vi "Do Obstacle Avoidance.vi"(5 "Target Distance":dbl=250.0, 8 "Wall Left?":bool=TRUE, 10 "Bot Angle (rad)":dbl=0.024476546476243494, 11 "Lidar Data (mm, rad)":cluster{dbl[], dbl[]}(graph)={[259.0, 261.0, 264.0, 264.0, 264.0, 261.0, 258.0, 258.0, 254.99999999999997, 255.0, 255.0, 253.0, 252.99999999999997, 260.0, 260.0, 260.0, 260.0, 260.0, 260.0, 257.0, 260.0, 263.0, 263.0, 262.0, 262.0, 260.0, 260.0, 262.0, 260.0, 263.0, 263.0, 256.0, 255.99999999999997, 256.0, 256.0, 260.0, 262.0, 262.0, 264.99999999999994, 262.0, 265.0, 265.0, 265.0, 265.0, 265.0, 265.0, 262.0, 262.0, 266.0, 266.0, 266.0, 266.0, 261.0, 259.0, 259.0, 259.0, 259.0, 261.0, 264.0, 261.0, 262.0, 262.0, 260.0, 260.0, 262.0, 262.0, 262.0, 262.0, 264.0, 263.0, 263.0, 272.0, 272.0, 272.0, 272.0, 272.0, 272.0, 272.0, 272.0, 272.0, 271.0, 270.0, 270.0, 269.0, 269.0, 269.0, 275.0, 276.0, 276.0, 277.0, 275.0, 277.0, 277.0, 277.0, 281.0, 281.0, 281.0, 284.0, 281.0, 281.0, 282.0, 282.0, 282.0, 283.0, 283.0, 295.99999999999994, 296.0, 291.00000000000006, 291.0, 291.0, 290.0, 291.0, 291.0, 291.0, 291.0, 300.0, 299.0, 299.0, 300.0, 307.0, 304.0, 311.0, 311.0, 308.0, 308.0, 308.0, 308.0, 308.0, 313.0, 319.0, 319.0, 322.0, 323.0, 326.0, 324.0, 326.0, 326.0, 329.0, 331.0, 336.99999999999994, 338.0, 338.0, 338.0, 338.0, 338.0, 338.0, 345.00000000000006, 350.0, 348.0, 349.99999999999994, 350.0, 351.0, 355.0, 358.0, 358.99999999999994, 358.0, 359.0, 367.0, 370.0, 367.00000000000006, 370.0, 372.0, 379.0, 379.0, 385.0, 387.0, 388.0, 394.0, 406.0, 406.99999999999994, 407.0, 408.0, 417.00000000000006, 417.0, 417.0, 417.0, 424.0, 428.0, 427.99999999999994, 428.99999999999994, 432.0, 432.0, 443.00000000000006, 452.0, 452.0, 454.0, 462.0, 464.00000000000006, 464.0, 464.00000000000006, 470.0, 480.99999999999994, 484.0, 494.0, 498.00000000000006, 499.00000000000006, 509.00000000000006, 508.99999999999994, 514.0, 521.0, 522.0, 533.0, 545.0, 546.0, 551.0, 555.0, 557.0, 567.0, 570.0, 573.0, 595.0, 606.0, 617.0, 619.0, 638.0, 643.0, 650.0, 667.0, 734.0, 734.0, 733.9999999999999, 728.0000000000001, 725.0, 720.0, 716.0, 713.0000000000001, 713.0, 715.0, 715.0, 714.9999999999999, 715.0, 698.0, 698.0, 698.0, 699.0000000000001, 699.0, 699.0, 693.0, 693.0, 693.0, 697.0, 697.0, 697.0, 688.0, 685.0, 684.9999999999999, 680.0, 684.0, 684.0, 684.0, 675.0, 683.0, 680.0, 680.0, 671.0, 670.0, 668.0, 667.9999999999999, 668.0, 668.0, 662.0, 668.0, 668.0, 669.9999999999999, 670.0, 670.0, 660.0, 659.0, 659.0, 660.0, 660.0, 662.0, 662.0, 661.0, 661.0, 661.0, 655.0, 655.0, 655.0, 653.0, 655.0, 654.0, 666.0, 654.0, 666.0, 654.0, 653.0, 647.0, 647.0, 647.0, 647.0, 651.0, 652.0, 653.0, 654.0, 654.0, 654.0, 654.0, 648.0, 648.0, 654.0, 650.0, 657.0, 657.0, 656.0, 654.0, 656.0, 656.0, 656.0, 654.0, 654.0, 654.0, 654.0, 654.0, 656.0, 656.0, 658.0, 656.0, 658.0, 656.0, 653.0, 650.0, 653.0, 652.9999999999999, 653.0, 659.0, 666.0, 666.0, 666.0000000000001, 670.0, 670.0, 670.0, 669.0000000000001, 670.0, 669.0, 670.0, 670.0, 678.0, 671.9999999999999, 678.0, 674.0, 678.0000000000001, 677.0, 683.0, 677.0, 677.0, 677.0, 688.0, 710.0, 782.0, 880.9999999999999, 840.0, 881.0, 881.0, 817.0, 896.0, 848.0, 848.0, 827.0, 815.0, 748.0, 748.0, 748.0, 754.0, 756.0, 68.0, 68.0, 68.0], [-1.7446474827552692, -1.7385115596037266, -1.732375636452184, -1.7262397133006415, -1.7201037901490988, -1.7139678669975562, -1.7078319438460137, -1.7016960206944711, -1.6955600975429286, -1.689424174391386, -1.6832882512398435, -1.677152328088301, -1.6710164049367584, -1.6648804817852159, -1.658744558633673, -1.6526086354821306, -1.646472712330588, -1.6403367891790455, -1.634200866027503, -1.6280649428759604, -1.6219290197244178, -1.6157930965728753, -1.6096571734213327, -1.6035212502697902, -1.5973853271182477, -1.591249403966705, -1.5851134808151623, -1.5789775576636198, -1.5728416345120773, -1.566705711360535, -1.5605697882089924, -1.5544338650574498, -1.5482979419059073, -1.5421620187543645, -1.536026095602822, -1.5298901724512795, -1.523754249299737, -1.5176183261481944, -1.5114824029966518, -1.5053464798451093, -1.4992105566935667, -1.4930746335420242, -1.4869387103904816, -1.480802787238939, -1.4746668640873963, -1.4685309409358538, -1.4623950177843112, -1.4562590946327687, -1.4501231714812262, -1.4439872483296836, -1.437851325178141, -1.4317154020265985, -1.425579478875056, -1.4194435557235134, -1.413307632571971, -1.4071717094204281, -1.4010357862688856, -1.394899863117343, -1.3887639399658005, -1.382628016814258, -1.3764920936627154, -1.3703561705111729, -1.3642202473596303, -1.3580843242080878, -1.3519484010565452, -1.3458124779050025, -1.33967655475346, -1.3335406316019174, -1.3274047084503748, -1.3212687852988323, -1.3151328621472897, -1.3089969389957472, -1.3028610158442047, -1.2967250926926621, -1.2905891695411196, -1.284453246389577, -1.2783173232380343, -1.2721814000864917, -1.2660454769349492, -1.2599095537834066, -1.253773630631864, -1.2476377074803215, -1.241501784328779, -1.2353658611772365, -1.229229938025694, -1.2230940148741514, -1.2169580917226088, -1.210822168571066, -1.2046862454195235, -1.198550322267981, -1.1924143991164384, -1.1862784759648959, -1.1801425528133533, -1.1740066296618108, -1.1678707065102683, -1.1617347833587257, -1.1555988602071832, -1.1494629370556404, -1.1433270139040979, -1.1371910907525553, -1.1310551676010128, -1.1249192444494702, -1.1187833212979277, -1.1126473981463851, -1.1065114749948426, -1.1003755518433, -1.0942396286917575, -1.088103705540215, -1.0819677823886722, -1.0758318592371297, -1.069695936085587, -1.0635600129340446, -1.057424089782502, -1.0512881666309595, -1.045152243479417, -1.0390163203278744, -1.0328803971763318, -1.0267444740247893, -1.0206085508732468, -1.014472627721704, -1.0083367045701614, -1.002200781418619, -0.9960648582670764, -0.9899289351155338, -0.9837930119639913, -0.9776570888124487, -0.9715211656609062, -0.9653852425093635, -0.959249319357821, -0.9531133962062782, -0.9469774730547359, -0.9408415499031934, -0.9347056267516507, -0.9285697036001082, -0.9224337804485656, -0.9162978572970231, -0.9101619341454805, -0.9040260109939379, -0.8978900878423952, -0.8917541646908528, -0.8856182415393102, -0.8794823183877678, -0.8733463952362251, -0.8672104720846825, -0.8610745489331402, -0.8549386257815974, -0.8488027026300549, -0.8426667794785123, -0.8365308563269697, -0.8303949331754271, -0.8242590100238846, -0.818123086872342, -0.8119871637207995, -0.8058512405692568, -0.7997153174177143, -0.793579394266172, -0.7874434711146292, -0.7813075479630864, -0.775171624811544, -0.7690357016600015, -0.7628997785084586, -0.7567638553569163, -0.7506279322053737, -0.7444920090538312, -0.7383560859022886, -0.732220162750746, -0.7260842395992034, -0.7199483164476609, -0.7138123932961183, -0.7076764701445758, -0.7015405469930333, -0.6954046238414906, -0.689268700689948, -0.6831327775384055, -0.676996854386863, -0.6708609312353204, -0.6647250080837778, -0.6585890849322352, -0.6524531617806927, -0.64631723862915, -0.6401813154776076, -0.6340453923260647, -0.6279094691745224, -0.6217735460229799, -0.6156376228714373, -0.6095016997198948, -0.6033657765683523, -0.5972298534168096, -0.591093930265267, -0.5849580071137245, -0.5788220839621819, -0.5726861608106395, -0.5665502376590967, -0.5604143145075542, -0.5542783913560116, -0.5481424682044691, -0.5420065450529266, -0.5358706219013839, -0.5297346987498412, -0.5235987755982987, -0.5174628524467563, -0.5113269292952137, -0.5051910061436712, -0.4990550829921286, -0.492919159840586, -0.48678323668904344, -0.4806473135375009, -0.47451139038595824, -0.46837546723441575, -0.4622395440828731, -0.4561036209313306, -0.44996769777978807, -0.44383177462824547, -0.4376958514767028, -0.43155992832516044, -0.4254240051736178, -0.41928808202207524, -0.4131521588705326, -0.4070162357189901, -0.40088031256744755, -0.39474438941590495, -0.38860846626436246, -0.38247254311281986, -0.3763366199612773, -0.3702006968097348, -0.3640647736581921, -0.35792885050664963, -0.351792927355107, -0.3456570042035645, -0.33952108105202194, -0.3333851579004794, -0.3272492347489368, -0.32111331159739426, -0.31497738844585166, -0.3088414652943091, -0.3027055421427665, -0.29656961899122397, -0.2904336958396814, -0.2842977726881388, -0.2781618495365963, -0.27202592638505374, -0.2658900032335112, -0.2597540800819686, -0.25361815693042605, -0.2474822337788835, -0.24134631062734088, -0.23521038747579834, -0.2290744643242557, -0.2229385411727132, -0.21680261802117062, -0.21066669486962808, -0.2045307717180855, -0.19839484856654294, -0.19225892541500036, -0.1861230022634578, -0.17998707911191522, -0.17385115596037265, -0.16771523280883013, -0.16157930965728756, -0.15544338650574496, -0.14930746335420234, -0.14317154020265982, -0.13703561705111728, -0.1308996938995747, -0.12476377074803216, -0.11862784759648957, -0.11249192444494702, -0.10635600129340447, -0.10022007814186189, -0.09408415499031934, -0.08794823183877676, -0.0818123086872342, -0.07567638553569163, -0.06954046238414907, -0.06340453923260649, -0.05726861608106395, -0.05113269292952138, -0.044996769777978805, -0.03886084662643624, -0.03272492347489367, -0.026589000323351118, -0.02045307717180855, -0.014317154020265985, -0.008181230868723419, -0.0020453077171808547, 0.0040906154343617095, 0.010226538585904275, 0.016362461737446838, 0.022498384888989403, 0.028634308040531974, 0.03477023119207454, 0.0409061543436171, 0.04704207749515967, 0.053178000646702236, 0.0593139237982448, 0.06544984694978735, 0.07158577010132992, 0.07772169325287247, 0.08385761640441505, 0.08999353955595761, 0.09612946270750018, 0.10226538585904273, 0.10840130901058531, 0.11453723216212788, 0.12067315531367044, 0.126809078465213, 0.13294500161675557, 0.13908092476829814, 0.1452168479198407, 0.15135277107138329, 0.15748869422292583, 0.1636246173744684, 0.16976054052601097, 0.1758964636775535, 0.1820323868290961, 0.18816830998063866, 0.19430423313218123, 0.20044015628372377, 0.20657607943526632, 0.2127120025868089, 0.21884792573835146, 0.22498384888989406, 0.23111977204143658, 0.23725569519297915, 0.24339161834452172, 0.24952754149606432, 0.25566346464760686, 0.2617993877991494, 0.2679353109506919, 0.2740712341022345, 0.2802071572537771, 0.2863430804053197, 0.2924790035568622, 0.2986149267084048, 0.30475084985994744, 0.3108867730114899, 0.31702269616303236, 0.32315861931457507, 0.3292945424661176, 0.33543046561766016, 0.34156638876920276, 0.3477023119207453, 0.3538382350722879, 0.35997415822383044, 0.366110081375373, 0.3722460045269156, 0.37838192767845813, 0.3845178508300008, 0.3906537739815433, 0.3967896971330859, 0.8017606251348951, 0.8078965482864374, 0.8140324714379802, 0.8201683945895226, 0.8263043177410653, 0.8324402408926079, 0.8508480103472355, 0.856983933498778, 0.8631198566503209, 0.8692557798018633, 0.8753917029534058, 0.8815276261049484, 0.8876635492564908, 0.8937994724080335, 0.8999353955595761, 1.6669257895023968, 1.6730617126539393, 1.679197635805482]}) -> (0 "Target Angle":dbl=0.040223878073184685)   [LabVIEW 2017]
uses:
  Globals/Pose.vi
  <vilib>/robotics/Obstacle Avoidance/Advanced Vector Field Histogram/NI_Robotics_Vector Field Histogram.lvlib
panel:
  in  "Max LIDAR Point Distance":dbl=4000.0 format="%#_13g"
  in  "Obstacle Clearance Distance":dbl=100.0 format="%#_13g"
  in  "VFH Threshold Distances":T1={"inner threshold distance"=350.0, "outer threshold distance"=360.0}
  out "LIDAR Data with Fake Wall":cluster{dbl[], dbl[]}(graph)
  # "Outputs"
  # "Inputs"
  # "Process"
  # "Thresholds need to be low enough to\nnot avoid the ramp before seeing red line"
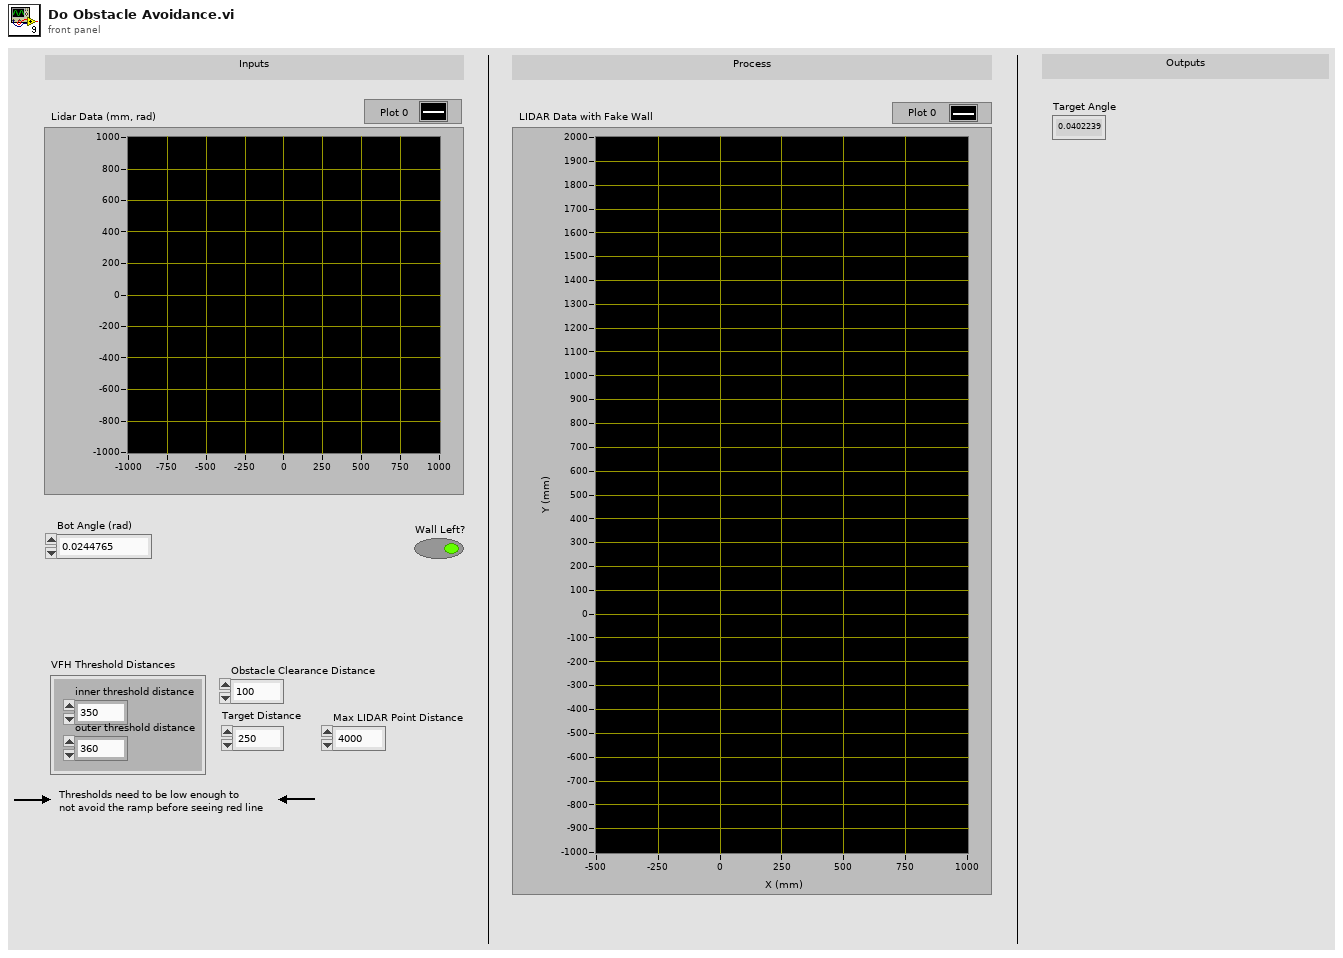
[diagram p1: front panel]
types:
  T1 = cluster{"inner threshold distance":dbl, "outer threshold distance":dbl}
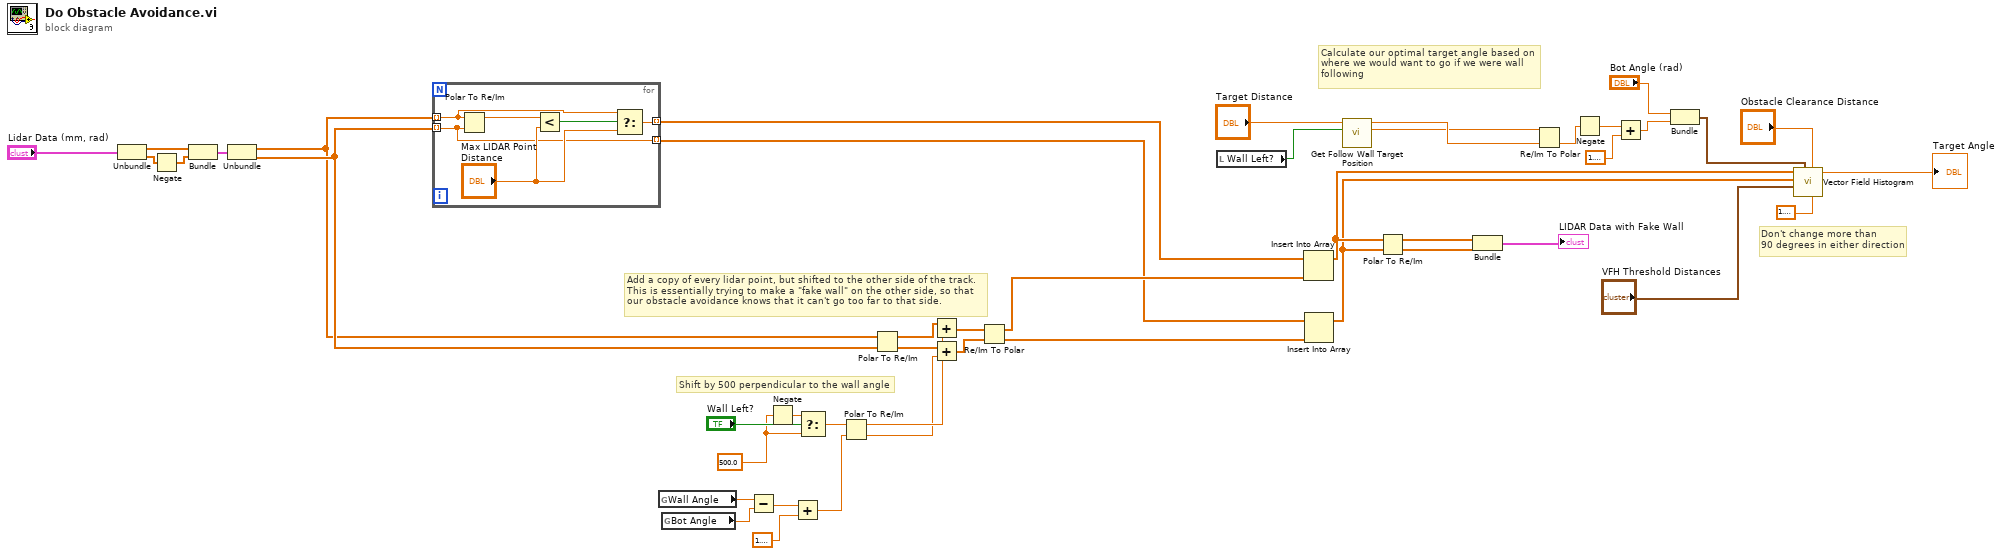
[diagram p0: block diagram]
diagram:
  w14 = 500.0 ("y")
  # "Shift by 500 perpendicular to the wall angle"
  # "Calculate our optimal target angle based on\nwhere we would want to go if we were wall\nfollowing"
  # "Don't change more than\n90 degrees in either direction"
  # "Add a copy of every lidar point, but shifted to the other side of the track.\nThis is essentially trying to make a \"fake wall\" on the other side, so that\nour obstacle avoidance knows that it can't go too far to that side."
  n1 = Unbundle("Lidar Data (mm, rad)") -> (w41:dbl[], w32:dbl[])
  n2 = Negate(x=w32) -> (-x=w31:dbl[])
  n3 = Bundle(w41, w31) -> (w40:cluster{dbl[], dbl[]})  [unwired: 1 in]
  n4 = Unbundle(w40) -> (w18:dbl[], w19:dbl[])
  n5 = for {
    tunnel: [w49] -> w20 mode=indexing
    tunnel: w19 -> [w46] mode=indexing
    tunnel: w18 -> [w47] mode=indexing
    tunnel: [w46] -> w16 mode=indexing
    n6 = Polar To Re/Im(2:w46, 3:w47) -> (1:w51:dbl)  [unwired: 1 out]
    n7 = Less?(x=w51, y="Max LIDAR Point Distance") -> (x < y?=w50:bool)
    n8 = Select(t=w47, s=w50, f="Max LIDAR Point Distance") -> (s? t:f=w49:dbl)
  }
  n9 = global read "Pose.vi" "Wall Angle"() -> (w5:dbl)
  n10 = global read "Pose.vi" "Bot Angle"() -> (w4:dbl)
  n11 = Subtract(x=w5, y=w4) -> (x-y=w3:dbl)
  n12 = Negate(x=w14) -> (-x=w21:dbl)
  n13 = Add(x=w3, y=1.5707963267948966) -> (x+y=w1:dbl)
  n14 = Select(t=w21, s="Wall Left?", f=w14) -> (s? t:f=w11:dbl)
  n15 = Polar To Re/Im(2:w1, 3:w11) -> (0:w6:dbl, 1:w7:dbl)
  n16 = Polar To Re/Im(2:w19, 3:w18) -> (0:w24:dbl[], 1:w8:dbl[])
  n17 = Add(x=w8, y=w7) -> (x+y=w9:dbl[])
  n18 = Add(x=w24, y=w6) -> (x+y=w10:dbl[])
  n19 = Re/Im To Polar(2:w10, 3:w9) -> (0:w22:dbl[], 1:w23:dbl[])
  n20 = local read "Wall Left?"() -> (w15:bool)
  n21 = Insert Into Array(array=w20, new element=w23) -> (w34:dbl[])  [unwired: 1 in]
  n22 = Insert Into Array(array=w16, new element=w22) -> (w33:dbl[])  [unwired: 1 in]
  n23 = call "Get Follow Wall Target Position.vi"("Wall left?"=w15, "Target Distance"="Target Distance") -> ("Target Y (Relative)"=w29:dbl, "Target X (Relative)"=w30:dbl)  [unwired: 6 in]
  n24 = Polar To Re/Im(2:w33, 3:w34) -> (0:w36:dbl[], 1:w37:dbl[])
  n25 = Bundle(w37, w36) -> (→"LIDAR Data with Fake Wall":cluster{dbl[], dbl[]})  [unwired: 1 in]
  n26 = Re/Im To Polar(2:w30, 3:w29) -> (0:w25:dbl)  [unwired: 1 out]
  n27 = Negate(x=w25) -> (-x=w26:dbl)
  n28 = Add(x=w26, y=1.5707963267948966) -> (x+y=w27:dbl)
  n29 = Bundle("Bot Angle (rad)"="Bot Angle (rad)", w27) -> (w44:cluster{"Bot Angle (rad)":dbl, dbl})  [unwired: 1 in]
  n30 = call <vilib>:"Vector Field Histogram.vi"("maximum heading change (rad)"=1.5707963267948966, "obstacle clearance distance"="Obstacle Clearance Distance", "heading"=w44, "thresholds"="VFH Threshold Distances", "direction angles (rad)"=w33, "distances"=w34) -> ("chosen heading (rad)"=→"Target Angle":dbl)  [unwired: 2 in, 3 out]
